vi "WSVCAP SHL FPGA LL Manage Initial States.vi"(0 "Transfer Cluster In":T1={"Transaction"=enum."I2C-Read Data", "Write Byte"=0, "Write Bits Remaining"=0, "Read Bits Remaining"=0, "Read Bytes Remaining"=0, "Wait Ticks Remaining"=0, "Slave Address"=0, "Bytes to Read"=2, "Bytes to Write"=0, "Sub Address"=2, "Socket Mask"=0, "Write CMD Idx [0-95]"=0, "Write Bit Index [0-18]"=0, "CMD Delay (Ticks)"=0, "Commands per Cycle [1-96]"=0, "CMD Length [1-48]"=1, "Cycle Count"=2, "Cycle Mode"=TRUE, "Cycle CMD"=0, "Transaction Step"=enum."I2C Write - I:Send Slave Address", "Operation Step"=enum."I2C Send Slave Add - A: Send Start Sequence", "Procedure Step"=enum."I2C Start/Stop - 1: Set Clock Low", "Start Operation"=FALSE, "Start Procedure"=FALSE, "Procedure"=enum."I2C-Send Address Byte", "Wait Ticks"=2, "UUT Set (0/1)"=0} {"Cycle CMD" format="%08x"; "Socket Mask" format="%06x"}) -> (4 "Transfer Cluster Out":T1={"Transaction"=enum."I2C-Read Data", "Write Byte"=0, "Write Bits Remaining"=0, "Read Bits Remaining"=0, "Read Bytes Remaining"=0, "Wait Ticks Remaining"=0, "Slave Address"=0, "Bytes to Read"=2, "Bytes to Write"=0, "Sub Address"=2, "Socket Mask"=0, "Write CMD Idx [0-95]"=0, "Write Bit Index [0-18]"=0, "CMD Delay (Ticks)"=0, "Commands per Cycle [1-96]"=0, "CMD Length [1-48]"=1, "Cycle Count"=2, "Cycle Mode"=TRUE, "Cycle CMD"=0, "Transaction Step"=enum."I2C Write - I:Send Slave Address", "Operation Step"=enum."I2C Send Slave Add - A: Send Start Sequence", "Procedure Step"=enum."I2C Start/Stop - 1: Set Clock Low", "Start Operation"=FALSE, "Start Procedure"=FALSE, "Procedure"=enum."I2C-Send Address Byte", "Wait Ticks"=2, "UUT Set (0/1)"=0} {"Cycle CMD" format="%08x"; "Socket Mask" format="%06x"})   [LabVIEW 2017]
uses:
  Type Defs/WSVCAP SHL Transaction Cluster.ctl
  Type Defs/WSVCAP SHL Transaction Enum.ctl
  Type Defs/WSVCAP SHL Transaction Step Enum.ctl
  Type Defs/WSVCAP SHL Operation Step Enum.ctl
  Type Defs/WSVCAP SHL Procedure Step Enum.ctl
  Type Defs/WSVCAP SHL Procedure Enum.ctl
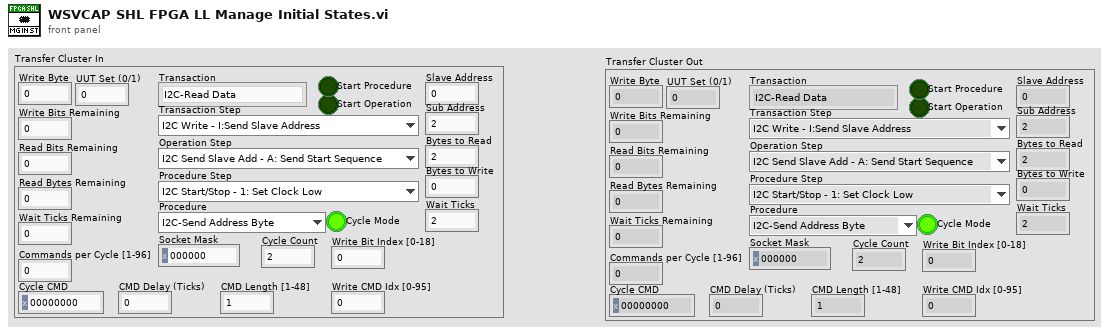
[diagram p1: front panel]
types:
  T1 = typedef "WSVCAP SHL Transaction Cluster.ctl" = cluster{"Transaction":T2, "Write Byte":u8, "Write Bits Remaining":u8, "Read Bits Remaining":u8, "Read Bytes Remaining":u8, "Wait Ticks Remaining":u32, "Slave Address":u8, "Bytes to Read":u8, "Bytes to Write":u8, "Sub Address":u8, "Socket Mask":u32, "Write CMD Idx [0-95]":u8, "Write Bit Index [0-18]":u8, "CMD Delay (Ticks)":u32, "Commands per Cycle [1-96]":u8, "CMD Length [1-48]":u8, "Cycle Count":u64, "Cycle Mode":bool, "Cycle CMD":u64, "Transaction Step":T3, "Operation Step":T4, "Procedure Step":T5, "Start Operation":bool, "Start Procedure":bool, "Procedure":T6, "Wait Ticks":u32, "UUT Set (0/1)":u8}
  T2 = typedef "WSVCAP SHL Transaction Enum.ctl" = enum16{"I2C-Read Data", "I2C-Write Data", "RFFE-Ext Write", "RFFE-Ext Read", "SRL-Write Data"}
  T3 = typedef "WSVCAP SHL Transaction Step Enum.ctl" = enum16{"I2C Write - I:Send Slave Address", "I2C Write - II:Send Sub Address", "I2C Write - III:Send Data Bytes", "I2C Read - I:Send Slave Address (W)", "I2C Read - II:Send Sub Address", "I2C Read - III:Send Slave Address (R)", "I2C Read - IV:Read Data Bytes", "RFFE Ext Write - I.Write Data", "RFFE Ext Read - I:Read Data", "SRL Write - I:Write Data"}
  T4 = typedef "WSVCAP SHL Operation Step Enum.ctl" = enum16{"I2C Send Slave Add - A: Send Start Sequence", "I2C Send Slave Add - B: Load Address Byte", "I2C Send Slave Add - C: Send Address Byte", "I2C Send Slave Add - D: Read Slave ACK", "I2C Send Sub Add - A: Load Sub Address", "I2C Send Sub Add - B: Send Address Byte", "I2C Send Sub Add - C: Read Slave ACK", "I2C Send Data - A: Get Byte from FIFO", "I2C Send Data - B: Send Data Byte", "I2C Send Data - C: Read Slave ACK", "I2C Send Data - D: Send Stop Sequence", "I2C Read Data - A: Load Bytes to Read", "I2C Read Data - B: Receive Byte", "I2C Read Data - C: Write Master ACK", "I2C Read Data - D: Send Stop Sequence", "RFFE Read Data - A: Send SSC", "RFFE Read Data - B: Send CMD Frame", "RFFE Read Data - C: Receive Byte", "RFFE Write Data - A: Send SSC", "RFFE Write Data - B: Send Data", "RFFE Write Data - C: Wait CMD Delay", "RFFE Write Data - D: Clear Lines", "SRL Write Data - A: Send Data", "SRL Write Data - B: Wait CMD Delay", "SRL Write Data - C: Clear Lines"}
  T5 = typedef "WSVCAP SHL Procedure Step Enum.ctl" = enum16{"I2C Start/Stop - 1: Set Clock Low", "I2C Start/Stop - 2: Wait", "I2C Start/Stop - 3: Set Data I", "I2C Start/Stop - 4: Wait", "I2C Start/Stop - 5: Set Clock High", "I2C Start/Stop - 6: Wait", "I2C Start/Stop - 7: Set Data II", "I2C Start/Stop - 8: Wait", "I2C Start/Stop - 9: Set Clock Low", "I2C Start/Stop - 10: Wait", "I2C Read ACK - 1: Set Clock High", "I2C Read ACK - 2: Wait", "I2C Read ACK - 3: Read ACK Bit", "I2C Read ACK - 4: Wait", "I2C Read ACK - 5: Set Clock Low", "I2C Read ACK - 6: Wait", "I2C Write ACK - 1: Write ACK Bit", "I2C Write ACK - 2: Wait", "I2C Write ACK - 3: Set Clock High", "I2C Write ACK - 4: Wait", "I2C Write ACK - 5: Set Clock Low", "I2C Write ACK - 6: Wait", "I2C Write ACK - 7: Set Data Low", "I2C Send Add - 1: Reset Bits Remaining", "I2C Send Add - 2: Set Data Bit", "I2C Send Add - 3: Wait", "I2C Send Add - 4: Set Clock High", "I2C Send Add - 5: Wait", "I2C Send Add - 6: Set Clock Low", "I2C Send Add - 7: Wait", "I2C Send Add - 8: Check Bits Remaining", "I2C Send Data - 1: Reset Bits Remaining", "I2C Send Data - 2: Load Write Bit from FIFO", "I2C Send Data - 3: Set Data Bit", "I2C Send Data - 4: Wait", "I2C Send Data - 5: Set Clock High", "I2C Send Data - 6: Wait", "I2C Send Data - 7: Set Clock Low", "I2C Send Data - 8: Wait", "I2C Send Data - 9: Check Bits Remaining", "I2C Receive Data - 1: Reset Bits Remaining", "I2C Receive Data - 2: Wait", "I2C Receive Data - 3: Set Clock High", "I2C Receive Data - 4: Wait", "I2C Receive Data - 5: Read Data Bit", "I2C Receive Data - 6: Wait", "I2C Receive Data - 7: Set Clock Low", "I2C Receive Data - 8: Wait", "I2C Receive Data - 9: Check Bits Remaining", "RFFE Send SSC - 1:Set Low", "RFFE Send SSC - 2:Wait", "RFFE Send SSC - 3:Set SDA High", "RFFE Send SSC - 4:Wait", "RFFE Send SSC - 5:Set SDA Low", "RFFE Send SSC - 6:Wait", "RFFE Send Data - 1:Set SCL High", "RFFE Send Data - 2:Wait", "RFFE Send Data - 3:Set SCL Low", "RFFE Send Data - 4:Wait", "RFFE Send Data - 5:Set SCL High (P)", "RFFE Send Data - 6:Wait", "RFFE Send Data - 7:Set SCL Low (P)", "RFFE Send Data - 8:Wait", "RFFE Send Data - 9:Set SCL High (BP)", "RFFE Send Data - 10:Wait", "RFFE Send Data - 11:Set SCL Low (BP)", "RFFE Send Data - 12:Wait", "RFFE Receive Data - 1:Set SCL High", "RFFE Receive Data - 2:Wait", "RFFE Receive Data - 3:Set SCL Low", "RFFE Receive Data - 4:Wait", "RFFE Receive Data - 5:Set SCL High (BP)", "RFFE Receive Data - 6:Wait", "RFFE Receive Data - 7:Set SCL Low (BP)", "RFFE Receive Data - 8:Wait", "RFFE Wait CMD Delay - 1:Wait", "RFFE Clear Lines - 1:Clear", "SRL Write Data - 1:Set SYNC High", "SRL Write Data - 2:Wait SYNC Delay", "SRL Write Data - 3:Set SYNC Low", "SRL Write Data - 4:Set SCLK High", "SRL Write Data - 5:Wait", "SRL Write Data - 6:Set SCLK Low", "SRL Write Data - 7:Wait", "SRL Write Data - 8:Set SYNC High", "SRL Wait CMD Delay - 1:Wait", "SRL Clear Lines - 1:Clear"}
  T6 = typedef "WSVCAP SHL Procedure Enum.ctl" = enum16{"None", "I2C-Send Start/Stop Sequence", "I2C-Send Address Byte", "I2C-Send Data Byte", "I2C-Read ACK", "I2C-Receive Byte", "I2C-Write ACK", "RFFE-Clear Lines", "RFFE-Send SSC", "RFFE-Send Data", "RFFE-Receive Data", "RFFE-Wait CMD Delay", "SRL-Clear Lines", "SRL-Send Data", "SRL-Wait CMD Delay"}
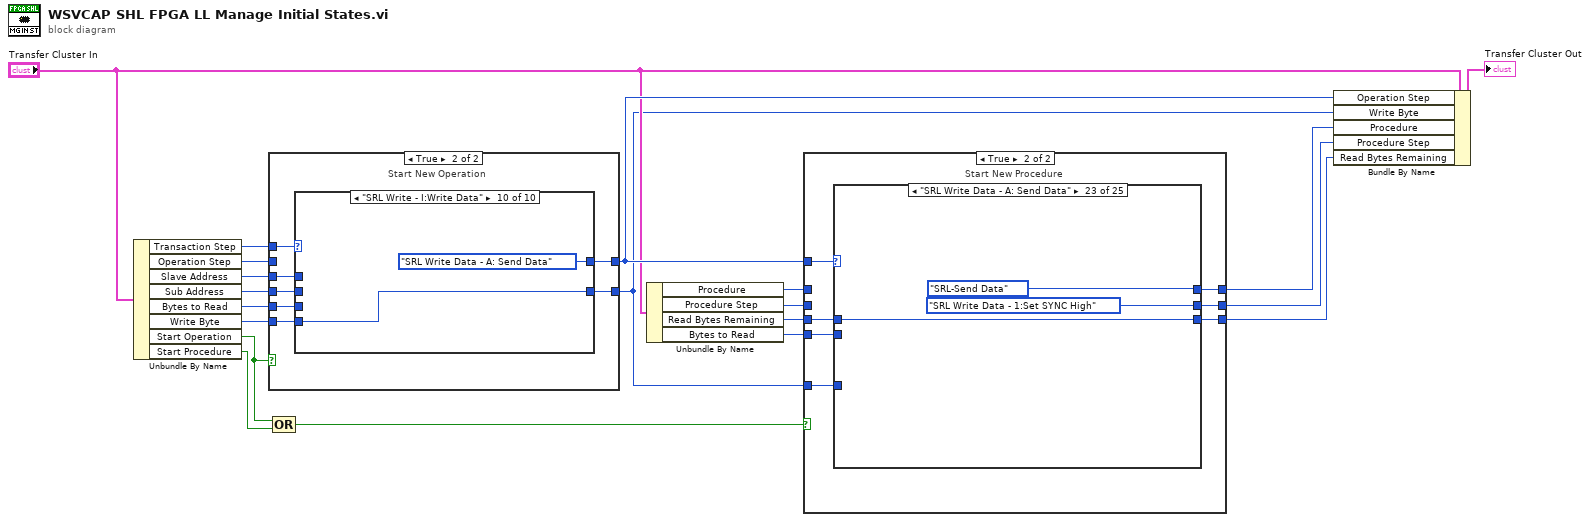
[diagram p0: block diagram]
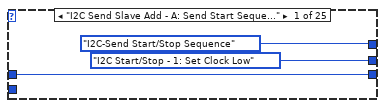
[diagram p3: hidden frame]
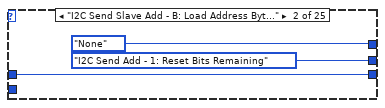
[diagram p4: hidden frame]
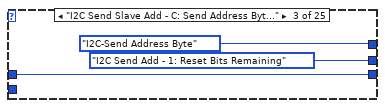
[diagram p5: hidden frame]
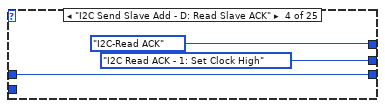
[diagram p6: hidden frame]
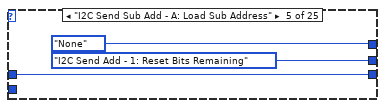
[diagram p7: hidden frame]
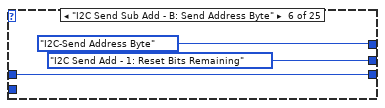
[diagram p8: hidden frame]
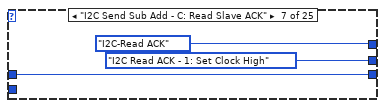
[diagram p9: hidden frame]
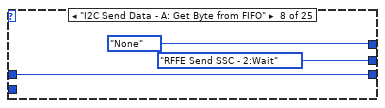
[diagram p10: hidden frame]
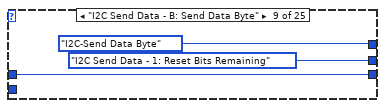
[diagram p11: hidden frame]
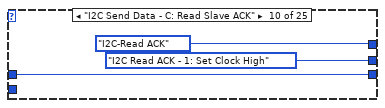
[diagram p12: hidden frame]
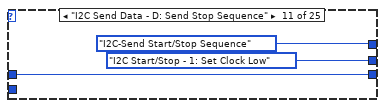
[diagram p13: hidden frame]
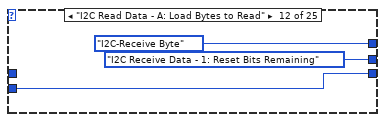
[diagram p14: hidden frame]
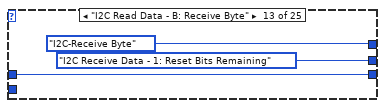
[diagram p15: hidden frame]
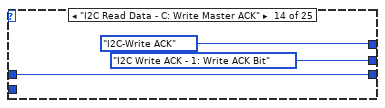
[diagram p16: hidden frame]
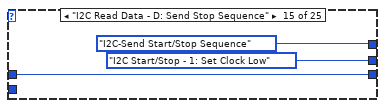
[diagram p17: hidden frame]
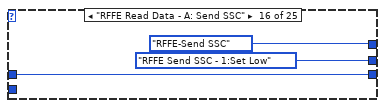
[diagram p18: hidden frame]
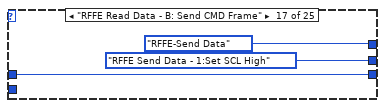
[diagram p19: hidden frame]
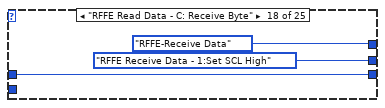
[diagram p20: hidden frame]
diagram:
  n1 = Unbundle By Name("Transfer Cluster In") -> ("Transaction Step"=w20:T3, "Operation Step"=w19:T4, "Slave Address"=w18:u8, "Sub Address"=w17:u8, "Bytes to Read"=w16:u8, "Write Byte"=w14:u8, "Start Operation"=w6:bool, "Start Procedure"=w5:bool)
  n2 = case shown="True" w6 {
    tunnel: w20 -> [_ w29]
    tunnel: [w22 w28] -> w13
    tunnel: w19 -> [w22 _]
    tunnel: w18 -> [_ w27]
    tunnel: w17 -> [_ w26]
    tunnel: w16 -> [_ w25]
    tunnel: [w21 w24] -> w1
    tunnel: w14 -> [w21 w23]
    frame False {
      # "Continue Current Operation"
    }
    frame True {
      # "Start New Operation"
      n3 = case shown="\"SRL Write - I:Write Data\"" w29 {
        tunnel: [WSVCAP_SHL_Operation_Step_Enum."I2C Send Slave Add - A: Send Start Sequence" ("Operation Step Out") WSVCAP_SHL_Operation_Step_Enum."I2C Send Sub Add - A: Load Sub Address" ("Operation Step Out") WSVCAP_SHL_Operation_Step_Enum."I2C Send Data - A: Get Byte from FIFO" ("Operation Step Out") WSVCAP_SHL_Operation_Step_Enum."I2C Send Slave Add - A: Send Start Sequence" ("Operation Step Out") WSVCAP_SHL_Operation_Step_Enum."I2C Send Sub Add - A: Load Sub Address" ("Operation Step Out") WSVCAP_SHL_Operation_Step_Enum."I2C Send Slave Add - A: Send Start Sequence" ("Operation Step Out") WSVCAP_SHL_Operation_Step_Enum."I2C Read Data - A: Load Bytes to Read" ("Operation Step Out") WSVCAP_SHL_Operation_Step_Enum."RFFE Write Data - A: Send SSC" ("Operation Step Out") WSVCAP_SHL_Operation_Step_Enum."RFFE Read Data - A: Send SSC" ("Operation Step Out") WSVCAP_SHL_Operation_Step_Enum."SRL Write Data - A: Send Data" ("Operation Step Out")] -> w28
        tunnel: w27 -> [w30 _ _ w36 _ w41 _ _ _ _]
        tunnel: w26 -> [_ w32 _ _ w38 _ _ _ _ _]
        tunnel: w25 -> [_ _ _ _ _ _ _ _ _ _]
        tunnel: [w30 w32 w34 w36 w38 w40 w44 w46 w48 w50] -> w24
        tunnel: w23 -> [_ _ w34 _ _ _ w44 w46 w48 w50]
        frame "I2C Write - I:Send Slave Address" {
        }
        frame "I2C Write - II:Send Sub Address" {
        }
        frame "I2C Write - III:Send Data Bytes" {
        }
        frame "I2C Read - I:Send Slave Address (W)" {
        }
        frame "I2C Read - II:Send Sub Address" {
        }
        frame "I2C Read - III:Send Slave Address (R)" {
          n4 = Compound Arithmetic op=OR(w41, u8 1 ("value")) -> (w40:u8)
        }
        frame "I2C Read - IV:Read Data Bytes" {
        }
        frame "RFFE Ext Write - I.Write Data" {
        }
        frame "RFFE Ext Read - I:Read Data" {
        }
        frame "SRL Write - I:Write Data" {
        }
      }
    }
  }
  n5 = Compound Arithmetic op=OR(w6, w5) -> (w15:bool)
  n6 = Unbundle By Name("Transfer Cluster In") -> ("Procedure"=w3:T6, "Procedure Step"=w12:T5, "Read Bytes Remaining"=w9:u8, "Bytes to Read"=w8:u8)
  n7 = case shown="True" w15 {
    tunnel: w13 -> [_ w61]
    tunnel: [w54 w60] -> w10
    tunnel: w12 -> [w54 _]
    tunnel: w9 -> [w53 w59]
    tunnel: w8 -> [_ w58]
    tunnel: [w53 w57] -> w7
    tunnel: [w52 w56] -> w2
    tunnel: w3 -> [w52 _]
    tunnel: w1 -> [_ w55]
    frame False {
      # "Continue Current Procedure"
    }
    frame True {
      # "Start New Procedure"
      n8 = case shown="\"SRL Write Data - A: Send Data\"" w61 {
        tunnel: [WSVCAP_SHL_Procedure_Step_Enum."I2C Start/Stop - 1: Set Clock Low" ("Procedure Step Out") WSVCAP_SHL_Procedure_Step_Enum."I2C Send Add - 1: Reset Bits Remaining" ("Procedure Step Out") WSVCAP_SHL_Procedure_Step_Enum."I2C Send Add - 1: Reset Bits Remaining" ("Procedure Step Out") WSVCAP_SHL_Procedure_Step_Enum."I2C Read ACK - 1: Set Clock High" ("Procedure Step Out") WSVCAP_SHL_Procedure_Step_Enum."I2C Send Add - 1: Reset Bits Remaining" ("Procedure Step Out") WSVCAP_SHL_Procedure_Step_Enum."I2C Send Add - 1: Reset Bits Remaining" ("Procedure Step Out") WSVCAP_SHL_Procedure_Step_Enum."I2C Read ACK - 1: Set Clock High" ("Procedure Step Out") WSVCAP_SHL_Procedure_Step_Enum."RFFE Send SSC - 2:Wait" ("Procedure Step Out") WSVCAP_SHL_Procedure_Step_Enum."I2C Send Data - 1: Reset Bits Remaining" ("Procedure Step Out") WSVCAP_SHL_Procedure_Step_Enum."I2C Read ACK - 1: Set Clock High" ("Procedure Step Out") WSVCAP_SHL_Procedure_Step_Enum."I2C Start/Stop - 1: Set Clock Low" ("Procedure Step Out") WSVCAP_SHL_Procedure_Step_Enum."I2C Receive Data - 1: Reset Bits Remaining" ("Procedure Step Out") WSVCAP_SHL_Procedure_Step_Enum."I2C Receive Data - 1: Reset Bits Remaining" ("Procedure Step Out") WSVCAP_SHL_Procedure_Step_Enum."I2C Write ACK - 1: Write ACK Bit" ("Procedure Step Out") WSVCAP_SHL_Procedure_Step_Enum."I2C Start/Stop - 1: Set Clock Low" ("Procedure Step Out") WSVCAP_SHL_Procedure_Step_Enum."RFFE Send SSC - 1:Set Low" ("Procedure Step Out") WSVCAP_SHL_Procedure_Step_Enum."RFFE Send Data - 1:Set SCL High" ("Procedure Step Out") WSVCAP_SHL_Procedure_Step_Enum."RFFE Receive Data - 1:Set SCL High" ("Procedure Step Out") WSVCAP_SHL_Procedure_Step_Enum."RFFE Send SSC - 1:Set Low" ("Procedure Step Out") WSVCAP_SHL_Procedure_Step_Enum."RFFE Send Data - 1:Set SCL High" ("Procedure Step Out") WSVCAP_SHL_Procedure_Step_Enum."RFFE Wait CMD Delay - 1:Wait" ("Procedure Step Out") WSVCAP_SHL_Procedure_Step_Enum."RFFE Clear Lines - 1:Clear" ("Procedure Step Out") WSVCAP_SHL_Procedure_Step_Enum."SRL Write Data - 1:Set SYNC High" ("Procedure Step Out") WSVCAP_SHL_Procedure_Step_Enum."SRL Wait CMD Delay - 1:Wait" ("Procedure Step Out") WSVCAP_SHL_Procedure_Step_Enum."SRL Clear Lines - 1:Clear" ("Procedure Step Out")] -> w60
        tunnel: [w63 w66 w69 w72 w75 w78 w81 w84 w87 w90 w93 w96 w99 w102 w105 w108 w111 w114 w117 w120 w123 w126 w129 w132 w135] -> w57
        tunnel: w59 -> [w63 w66 w69 w72 w75 w78 w81 w84 w87 w90 w93 _ w99 w102 w105 w108 w111 w114 w117 w120 w123 w126 w129 w132 w135]
        tunnel: w58 -> [_ _ _ _ _ _ _ _ _ _ _ w96 _ _ _ _ _ _ _ _ _ _ _ _ _]
        tunnel: [WSVCAP_SHL_Procedure_Enum."I2C-Send Start/Stop Sequence" ("Procedure") WSVCAP_SHL_Procedure_Enum."None" ("Procedure") WSVCAP_SHL_Procedure_Enum."I2C-Send Address Byte" ("Procedure") WSVCAP_SHL_Procedure_Enum."I2C-Read ACK" ("Procedure") WSVCAP_SHL_Procedure_Enum."None" ("Procedure") WSVCAP_SHL_Procedure_Enum."I2C-Send Address Byte" ("Procedure") WSVCAP_SHL_Procedure_Enum."I2C-Read ACK" ("Procedure") WSVCAP_SHL_Procedure_Enum."None" ("Procedure") WSVCAP_SHL_Procedure_Enum."I2C-Send Data Byte" ("Procedure") WSVCAP_SHL_Procedure_Enum."I2C-Read ACK" ("Procedure") WSVCAP_SHL_Procedure_Enum."I2C-Send Start/Stop Sequence" ("Procedure") WSVCAP_SHL_Procedure_Enum."I2C-Receive Byte" ("Procedure") WSVCAP_SHL_Procedure_Enum."I2C-Receive Byte" ("Procedure") WSVCAP_SHL_Procedure_Enum."I2C-Write ACK" ("Procedure") WSVCAP_SHL_Procedure_Enum."I2C-Send Start/Stop Sequence" ("Procedure") WSVCAP_SHL_Procedure_Enum."RFFE-Send SSC" ("Procedure") WSVCAP_SHL_Procedure_Enum."RFFE-Send Data" ("Procedure") WSVCAP_SHL_Procedure_Enum."RFFE-Receive Data" ("Procedure") WSVCAP_SHL_Procedure_Enum."RFFE-Send SSC" ("Procedure") WSVCAP_SHL_Procedure_Enum."RFFE-Send Data" ("Procedure") WSVCAP_SHL_Procedure_Enum."RFFE-Wait CMD Delay" ("Procedure") WSVCAP_SHL_Procedure_Enum."RFFE-Clear Lines" ("Procedure") WSVCAP_SHL_Procedure_Enum."SRL-Send Data" ("Procedure") WSVCAP_SHL_Procedure_Enum."SRL-Wait CMD Delay" ("Procedure") WSVCAP_SHL_Procedure_Enum."SRL-Clear Lines" ("Procedure")] -> w56
        tunnel: w55 -> [_ _ _ _ _ _ _ _ _ _ _ _ _ _ _ _ _ _ _ _ _ _ _ _ _]
        frame "I2C Send Slave Add - A: Send Start Sequence" {
        }
        frame "I2C Send Slave Add - B: Load Address Byte" {
        }
        frame "I2C Send Slave Add - C: Send Address Byte" {
        }
        frame "I2C Send Slave Add - D: Read Slave ACK" {
        }
        frame "I2C Send Sub Add - A: Load Sub Address" {
        }
        frame "I2C Send Sub Add - B: Send Address Byte" {
        }
        frame "I2C Send Sub Add - C: Read Slave ACK" {
        }
        frame "I2C Send Data - A: Get Byte from FIFO" {
        }
        frame "I2C Send Data - B: Send Data Byte" {
        }
        frame "I2C Send Data - C: Read Slave ACK" {
        }
        frame "I2C Send Data - D: Send Stop Sequence" {
        }
        frame "I2C Read Data - A: Load Bytes to Read" {
        }
        frame "I2C Read Data - B: Receive Byte" {
        }
        frame "I2C Read Data - C: Write Master ACK" {
        }
        frame "I2C Read Data - D: Send Stop Sequence" {
        }
        frame "RFFE Read Data - A: Send SSC" {
        }
        frame "RFFE Read Data - B: Send CMD Frame" {
        }
        frame "RFFE Read Data - C: Receive Byte" {
        }
        frame "RFFE Write Data - A: Send SSC" {
        }
        frame "RFFE Write Data - B: Send Data" {
        }
        frame "RFFE Write Data - C: Wait CMD Delay" {
        }
        frame "RFFE Write Data - D: Clear Lines" {
        }
        frame "SRL Write Data - A: Send Data" {
        }
        frame "SRL Write Data - B: Wait CMD Delay" {
        }
        frame "SRL Write Data - C: Clear Lines" {
        }
      }
    }
  }
  n9 = Bundle By Name(cluster="Transfer Cluster In", "Operation Step"=w13, "Write Byte"=w1, "Procedure"=w2, "Procedure Step"=w10, "Read Bytes Remaining"=w7) -> (→"Transfer Cluster Out":T1)
